vi "Move Selection.vi"   [LabVIEW 2023]
doc: "This example illustrates the Move Selected Objects method in VI Scripting, which programmatically triggers a mouse-drag in the editing environment. This can be a useful way to manipulate multiple objects.\n\nA Move operation can be made into a copy by specifying a 'Duplicate?' value of TRUE."
uses:
  <vilib>/Utility/miscctls.llb/LVDeltaXY32Cluster.ctl
panel:
  # "Overview: Demonstrates the Move Selected Objects method in VI Scripting, which moves the current selection to a different location.\nInstructions:\n1. Open the block diagram of Test - Selection List Target.vi.\n2. Select one or more objects.\n3. Run this VI. The selected objects will be moved up 25 pixels on the diagram."
types:
  T1 = typedef "LVDeltaXY32Cluster.ctl" = cluster{"X":i32, "Y":i32}
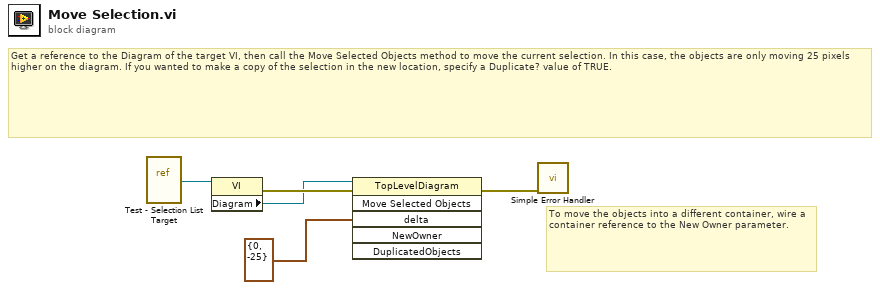
[diagram p0: block diagram]
diagram:
  # "Get a reference to the Diagram of the target VI, then call the Move Selected Objects method to move the current selection. In this case, the objects are only moving 25 pixels higher on the diagram. If you wanted to make a copy of the selection in the new location, specify a Duplicate? value of TRUE."
  # "To move the objects into a different container, wire a container reference to the New Owner parameter."
  n1 = vi-ref "Test - Selection List Target.vi"() -> (w5:refnum<vi>)
  n2 = property class="VI"(reference=w5) -> (error out=w3:errorcluster, "Diagram"=w2:refnum<vi>)  [unwired: 1 in, 1 out]
  n3 = invoke class="TopLevelDiagram" method="Move Selected Objects"(reference=w2, error in=w3, "delta"=T1 {"X"=0, "Y"=-25} ("X/Y Delta")) -> (error out=w1:errorcluster)  [unwired: 3 in, 5 out]
  n4 = call <vilib>:"Simple Error Handler.vi"("error in (no error)"=w1) -> ()  [unwired: 4 in, 5 out]
